vi "DKv_2024.vi"(0 "Temperature [K]":dbl=293.15 format="%.4f", 1 "Pressure [Pa]":dbl=101325.0 format="%.1f", 2 "Type of air":i32(listbox)=4, 3 "xw molar fraction of water vapor":dbl=0.015, 4 "CO2 content (ppm)":dbl=500.0) -> (5 "DKv":dbl=3.673306522180785e-05 format="%#.6f", 6 "Uv1":dbl=1.778191226882398, 7 "Uv2":dbl=2.8840142305300334e-05, 8 "DKv/1+Kv":dbl=3.671283343836786e-05, 9 "Uv3":dbl=2.3259472252997204, 10 "Kv":dbl=0.000551082048024398 format="%.6f")   [LabVIEW 2016]
panel:
  out "3rd vir contr to Kv":dbl format="%_3e"
  out "2nd vir contr to kV":dbl format="%.3e"
  out "DC / cm6 mol-2":dbl
  out "DCd / cm6 mol-2":dbl
  out "DCw / cm6 mol-2":dbl
  out "C / cm6 mol-2":dbl=-9.308026939937086
  out "Cw / cm6 mol-2":dbl=-9.308026939937086
  out "Cd / cm6 mol-2":dbl=-9.308026939937086
  out "DBdw / cm3 mol-1":dbl
  out "Bdw / cm3 mol-1":dbl=-9.308026939937086
  out "Bw / cm3 mol-1":dbl=-9.308026939937086
  out "Bd / cm3 mol-1":dbl=-9.308026939937086
  out "B / cm3 mol-1":dbl
  out "DBw / cm3 mol-1":dbl
  out "DBd / cm3 mol-1":dbl
  out "DB / cm3 mol-1":dbl
  # "±"
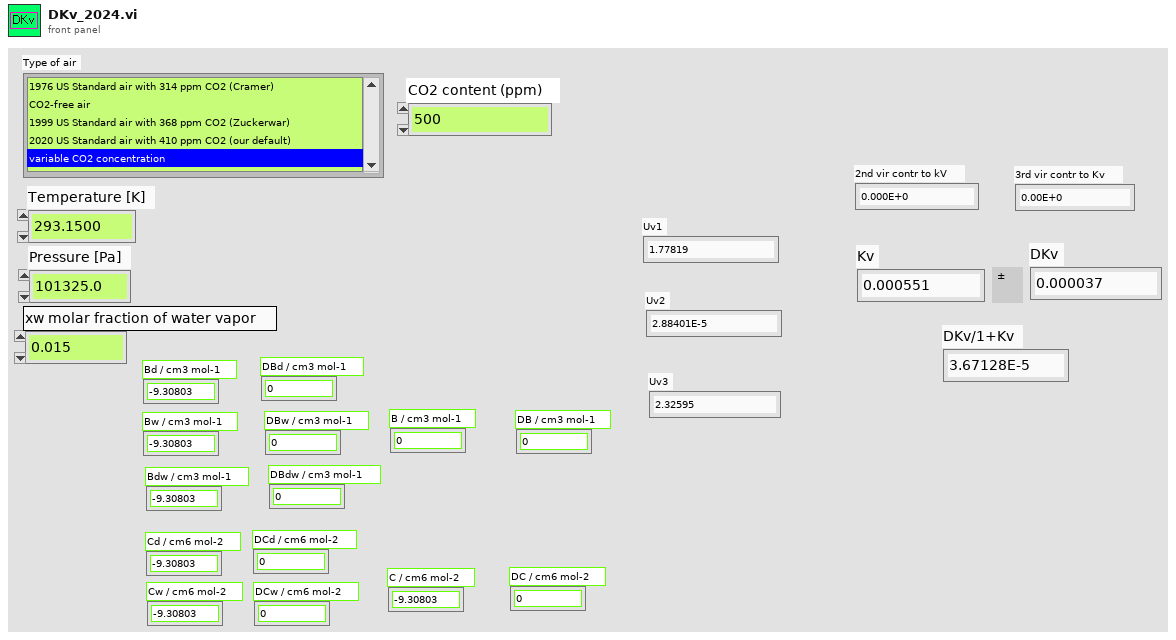
[diagram p1: front panel]
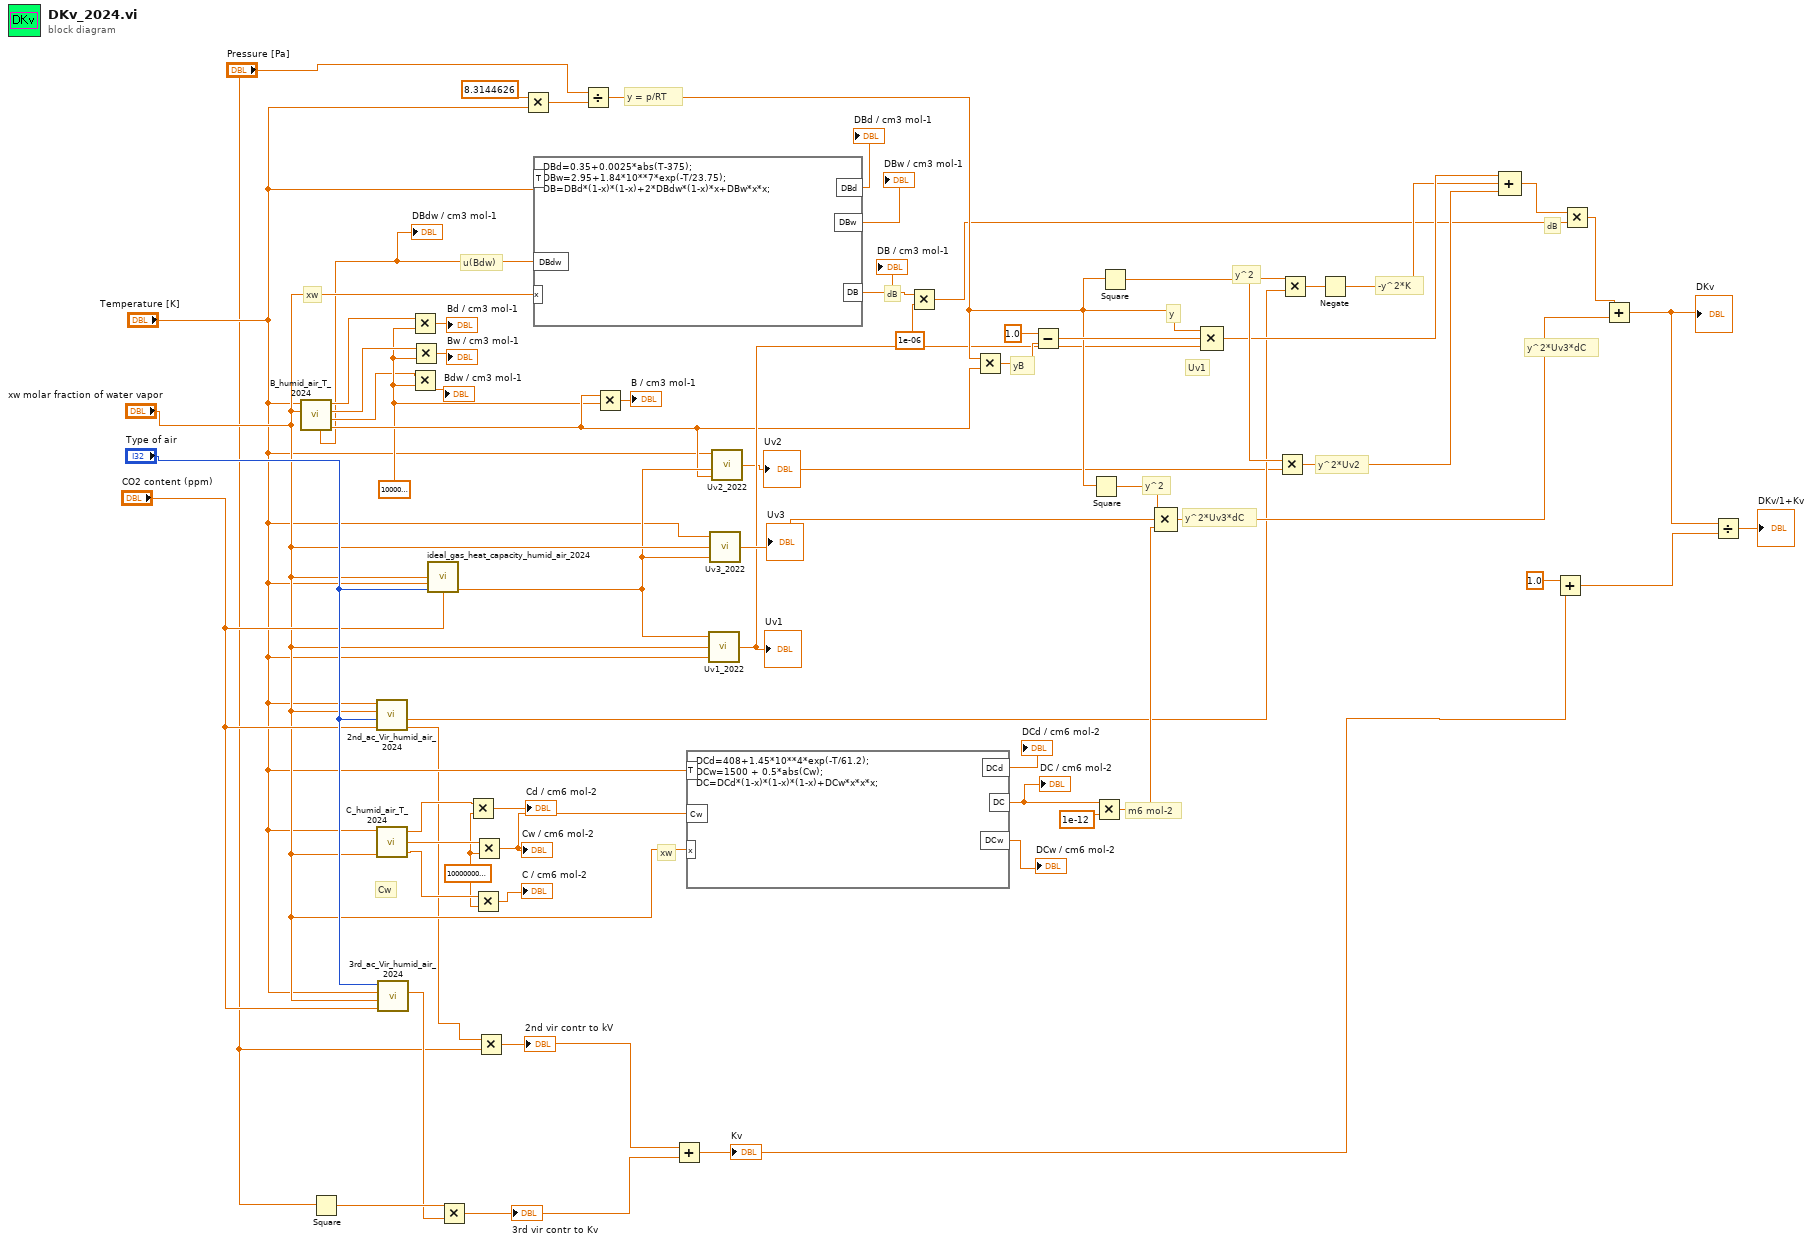
[diagram p0: block diagram]
diagram:
  w22 = 1000000.0 ("y")
  w14 = 1000000000000.0 ("y")
  # "xw"
  # "xw"
  # "m6 mol-2"
  # "Cw"
  # "u(Bdw)"
  # "y^2*Uv2"
  # "-y^2*K"
  # "y^2"
  # "dB"
  # "dB"
  # "y^2*Uv3*dC"
  # "y^2"
  # "y^2*Uv3*dC"
  # "Uv1"
  # "y"
  # "yB"
  # "y = p/RT"
  n1 = call "B_humid_air_T_2024.vi"("xw molar fraction water vapor"="xw molar fraction of water vapor", "Temperature (K)"="Temperature [K]") -> ("Bhumid air (xw,T) [m^3/mol]"=w30:dbl, "Bdw(T) [m^3/mol]"=w21:dbl, "Bw(T) [m^3/mol]"=w25:dbl, "Bd(T) [m^3/mol]"=w26:dbl, "u(Bdw) [cm^3/mol]"=w19:dbl)  [unwired: 5 in]
  "DBdw / cm3 mol-1" <- w19
  n2 = Square(x="Pressure [Pa]") -> (x^2=w7:dbl)
  n3 = call "2nd_ac_Vir_humid_air_2024.vi"("CO2 content (ppm)"="CO2 content (ppm)", "Type of air"="Type of air", "xw molar fraction water vapor"="xw molar fraction of water vapor", "Temperature (K)"="Temperature [K]") -> ("2nd ac pressure vir humid air b or \"F\""=w2:dbl, "2nd ac vir humid air \"K\""=w34:dbl)  [unwired: 2 out]
  n4 = call "C_humid_air_T_2024.vi"("xw molar fraction water vapor"="xw molar fraction of water vapor", "Temperature (K)"="Temperature [K]") -> ("C humid air [m^3/mol]^2"=w15:dbl, "C water (m^3/mol)^2"=w16:dbl, "C dryair (m^3/mol)^2"=w18:dbl)  [unwired: 2 in]
  n5 = call "3rd_ac_Vir_humid_air_2024.vi"("CO2 content (ppm)"="CO2 content (ppm)", "Water Vapor Mole Fraction"="xw molar fraction of water vapor", "Temperature [K]"="Temperature [K]", "Type of air"="Type of air") -> ("3rd ac press Virial [G]"=w4:dbl)  [unwired: 2 in, 5 out]
  n6 = Multiply(x=w26, y=w22) -> (x*y=→"Bd / cm3 mol-1":dbl)
  n7 = Multiply(x=w21, y=w22) -> (x*y=→"Bdw / cm3 mol-1":dbl)
  n8 = Multiply(x=w25, y=w22) -> (x*y=→"Bw / cm3 mol-1":dbl)
  n9 = call "ideal_gas_heat_capacity_humid_air_2024.vi"("molar fraction of water vapor"="xw molar fraction of water vapor", "Temperature [K]"="Temperature [K]", "Type of air"="Type of air", "CO2 content (ppm)"="CO2 content (ppm)") -> ("Gamma0 humid air"=w32:dbl)  [unwired: 2 in, 9 out]
  n10 = Multiply(x=w7, y=w4) -> (x*y=w5:dbl)
  "3rd vir contr to Kv" <- w5
  n11 = Multiply(x=w18, y=w14) -> (x*y=→"Cd / cm6 mol-2":dbl)
  n12 = Multiply(x=w15, y=w14) -> (x*y=→"C / cm6 mol-2":dbl)
  n13 = Multiply(x=w16, y=w14) -> (x*y=w8:dbl)
  "Cw / cm6 mol-2" <- w8
  n14 = Multiply(x=w2, y="Pressure [Pa]") -> (x*y=w6:dbl)
  "2nd vir contr to kV" <- w6
  n15 = Multiply(x=8.3144626, y="Temperature [K]") -> (x*y=w62:dbl)
  n16 = formula code="DBd=0.35+0.0025*abs(T-375);\nDBw=2.95+1.84*10**7*exp(-T/23.75);\nDB=DBd*(1-x)*(1-x)+2*DBdw*(1-x)*x+DBw*x*x;"("x"="xw molar fraction of water vapor", "T"="Temperature [K]", "DBdw"=w19) -> ("DB"=w41:dbl, "DBd"=→"DBd / cm3 mol-1":dbl, "DBw"=→"DBw / cm3 mol-1":dbl)
  "DB / cm3 mol-1" <- w41
  n17 = Divide(x="Pressure [Pa]", y=w62) -> (x/y=w44:dbl)
  n18 = Multiply(x=w30, y=w22) -> (x*y=→"B / cm3 mol-1":dbl)
  n19 = Add(x=w6, y=w5) -> (x+y=w1:dbl)
  "Kv" <- w1
  n20 = formula code="DCd=408+1.45*10**4*exp(-T/61.2);\nDCw=1500 + 0.5*abs(Cw);\nDC=DCd*(1-x)*(1-x)*(1-x)+DCw*x*x*x;"("x"="xw molar fraction of water vapor", "T"="Temperature [K]", "Cw"=w8) -> ("DC"=w10:dbl, "DCd"=→"DCd / cm6 mol-2":dbl, "DCw"=→"DCw / cm6 mol-2":dbl)
  "DC / cm6 mol-2" <- w10
  n21 = call "Uv1_2022.vi"("Temperature [K]"="Temperature [K]", "xw"="xw molar fraction of water vapor", "Gamma0 humid air"=w32) -> ("Uv1"=w35:dbl)
  "Uv1" <- w35
  n22 = call "Uv3_2022.vi"("Gamma0 humid air"=w32, "xw water mol fraction"="xw molar fraction of water vapor", "Temperature [K]"="Temperature [K]") -> ("Uv3"=w51:dbl)
  "Uv3" <- w51
  n23 = call "Uv2_2022.vi"("B(T)"=w30, "Gamma0 humid air"=w32, "Temperature [K]"="Temperature [K]") -> ("Uv2"=w31:dbl)  [unwired: 1 in]
  "Uv2" <- w31
  n24 = Multiply(x=w41, y=1e-06) -> (x*y=w36:dbl)
  n25 = Multiply(x=w44, y=w30) -> (x*y=w59:dbl)
  n26 = Subtract(x=1.0, y=w59) -> (x-y=w58:dbl)
  n27 = Square(x=w44) -> (x^2=w50:dbl)
  n28 = Multiply(x=w10, y=1e-12) -> (x*y=w42:dbl)
  n29 = Square(x=w44) -> (x^2=w57:dbl)
  n30 = Compound Arithmetic op=MULTIPLY(w50, w51, w42) -> (w48:dbl)
  n31 = Compound Arithmetic op=MULTIPLY(w44, w58, w35) -> (w56:dbl)
  n32 = Multiply(x=w57, y=w31) -> (x*y=w53:dbl)
  n33 = Multiply(x=w57, y=w34) -> (x*y=w55:dbl)
  n34 = Negate(x=w55) -> (-x=w54:dbl)
  n35 = Compound Arithmetic op=ADD(w56, w54, w53) -> (w52:dbl)
  n36 = Add(x=1.0, y=w1) -> (x+y=w46:dbl)
  n37 = Multiply(x=w52, y=w36) -> (x*y=w49:dbl)
  n38 = Add(x=w49, y=w48) -> (x+y=w33:dbl)
  "DKv" <- w33
  n39 = Divide(x=w33, y=w46) -> (x/y=→"DKv/1+Kv":dbl)
